vi "Global.vi"() -> ()   [LabVIEW 2010, in "RefMem PtByPt Custom Device.lvlib"]
uses:
  RefMem PtByPt Custom Device.lvlib
panel:
  out "CPU":string="CPU"
  out "Type":string="Type"
  out "Main Page GUID":string="7909965F-057A-768C-4F90-62AAAF60C660"
  out "Status Section GUID":string="F16F71FA-3FA0-97FC-1B57-1BD394F34D00"
  out "VISA Name":string="VISA Name"
  out "Address":string="Address"
  out "Del Prot Chan GUID":string="C857B30F-F7F9-BC70-992A-D64B2B0468D2"
  out "Data Channel GUID":string="9326A373-E05B-AEFA-6A61-3C021DFF52FF"
  out "Data Folder GUID":string="2F571347-8FFC-7952-DED1-8B6F86A612BB"
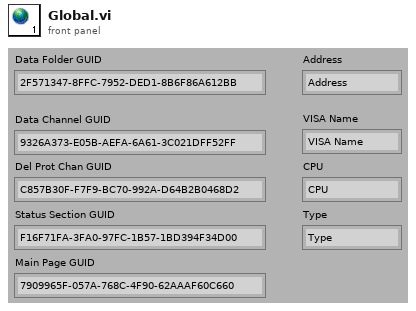
[diagram p1: front panel]
diagram:
